vi "hough transform.vi"(10 "Threshold (0 - 255)":u8) -> (0 "error out":errorcluster)   [LabVIEW 2012]
uses:
  <vilib>/vision/Image Controls.llb/IMAQ Image.ctl
  <vilib>/vision/NI_Vision_Development_Module.lvlib
panel:
  out "Numeric 2":u32
  out "Numeric":u32
  out "Image 3":T1(plugin-control)
  out "Image 2":T1(plugin-control)
  in  "error in":errorcluster
  out "Image":T1
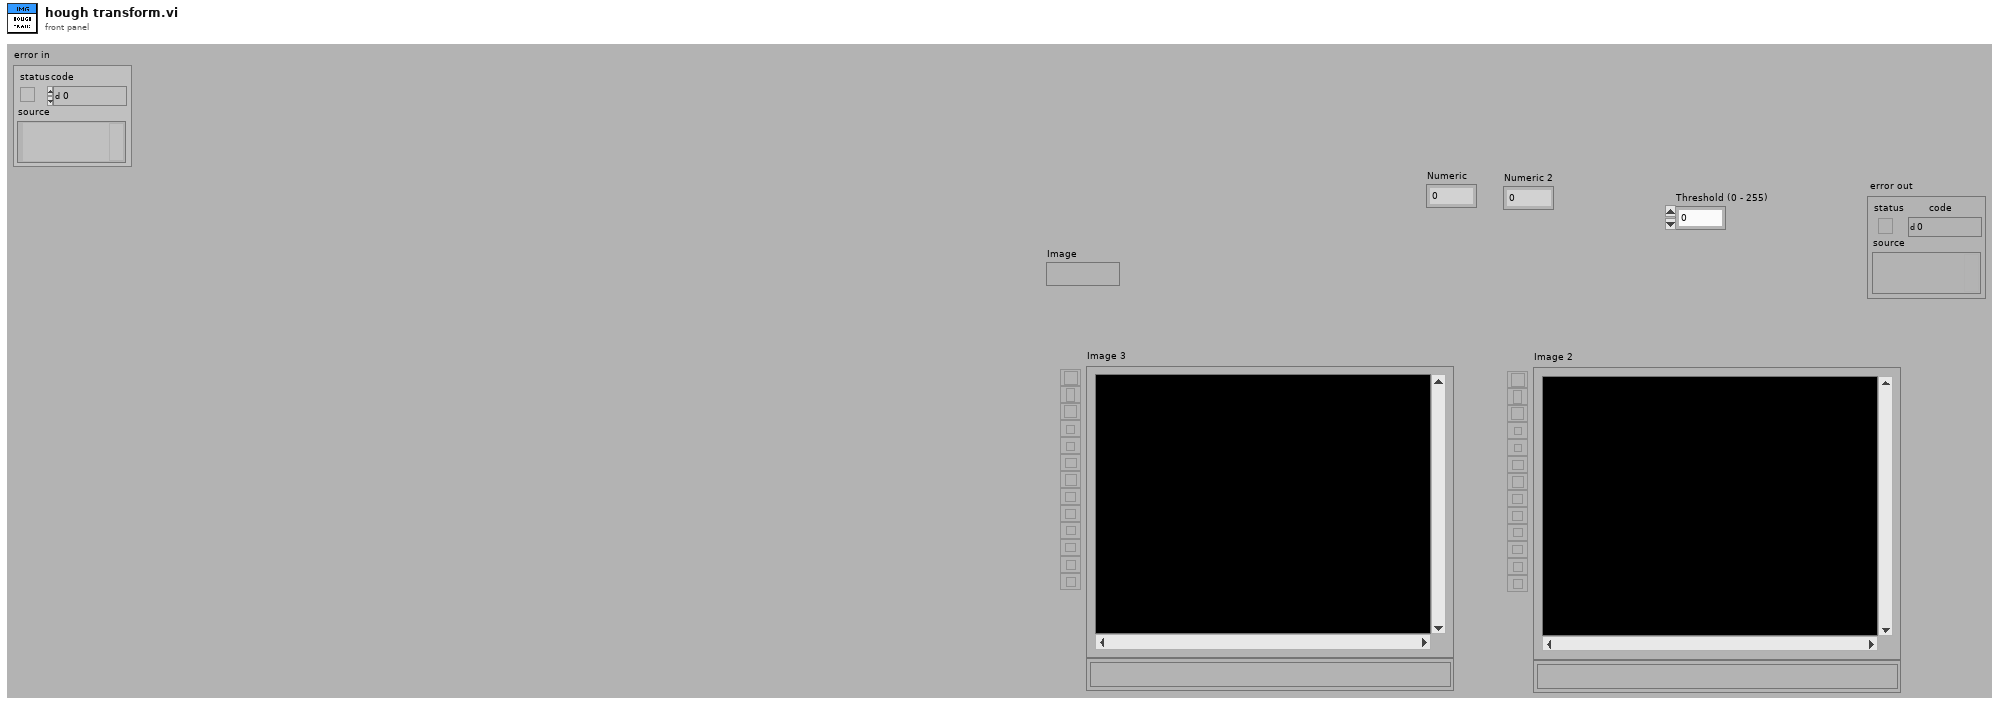
[diagram p1: front panel]
types:
  T1 = typedef "IMAQ Image.ctl" = refnum<image>
  T2 = typedef "Image Type" = u32
  T3 = enum32{"8 bits", "16 bits", "Float", "Complex", "RGB Chunky", "Compressed"}
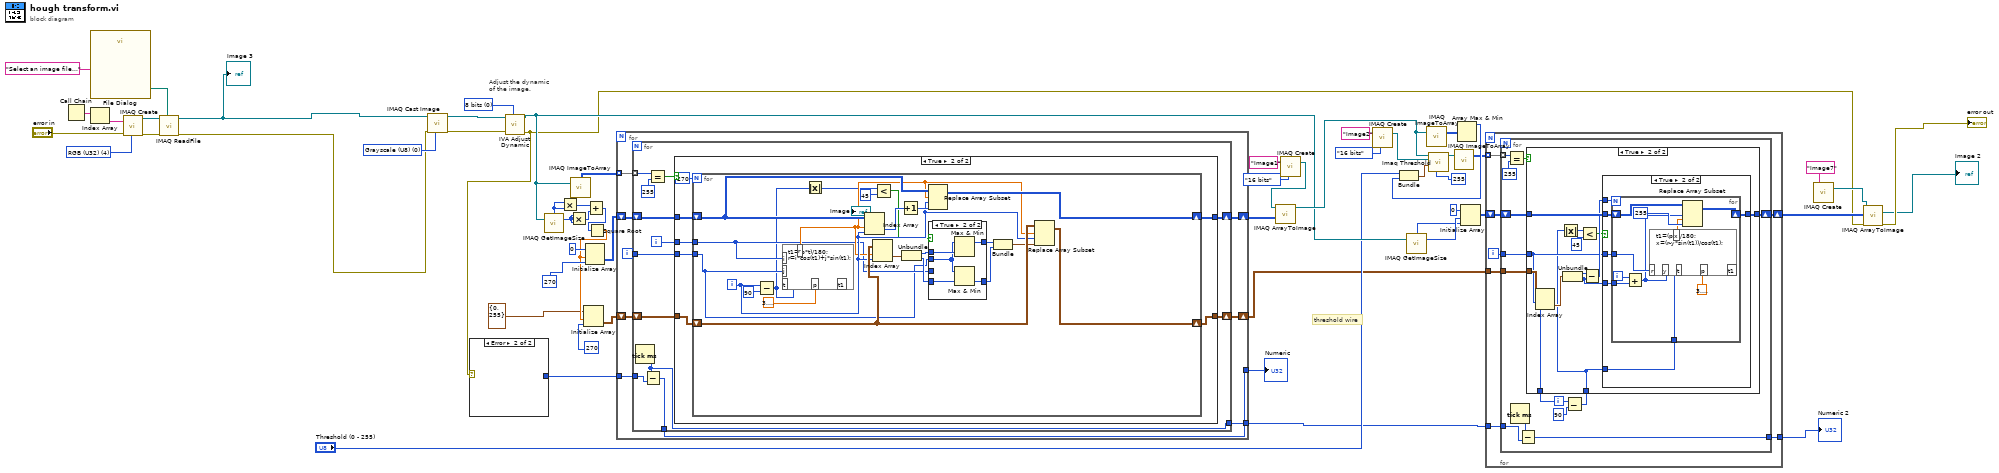
[diagram p0: block diagram]
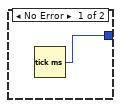
[diagram p2: hidden frame]
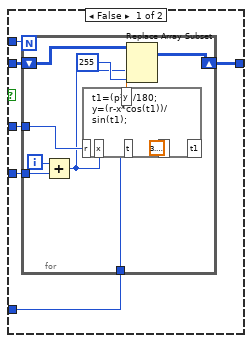
[diagram p4: hidden frame]
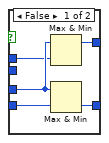
[diagram p6: hidden frame]
diagram:
  w10 = T2 4 items=["Grayscale (U8)", "Grayscale (I16)", "Grayscale (SGL)", "Complex (CSG)", "RGB (U32)", "HSL (U32)", "RGB (U64)", "Grayscale (U16)"] ("Image Type")
  w19 = T2 0 items=["Grayscale (U8)", "Grayscale (I16)", "Grayscale (SGL)", "Complex (CSG)", "RGB (U32)", "HSL (U32)", "RGB (U64)", "Grayscale (U16)"] ("Image Type")
  w24 = u32 0 items=["8 bits", "16 bits", "Float", "Complex", "RGB", "HSL"] ("Image Type")
  # "threshold wire"
  # "Adjust the dynamic\nof the image."
  n1 = Call Chain() -> (call chain=w14:string[])
  n2 = Index Array(array=w14) -> (element=w13:string)  [unwired: 1 in]
  n3 = call "File Dialog"("prompt"="Select an image file...") -> ("selected path"=w11:path)  [unwired: 6 in, 8 out]
  n4 = call "IMAQ Create"("Image Name"=w13, "Image Type"=w10, "error in (no error)"="error in") -> ("New Image"=w17:T1, "error out"=w16:errorcluster)  [unwired: 1 in, 1 out]
  n5 = call "IMAQ ReadFile"("File Path"=w11, "error in (no error)"=w16, "Image"=w17) -> ("error out"=w9:errorcluster, "Image Out"=w7:T1)  [unwired: 2 in, 5 out]
  "Image 3" <- w7
  n6 = call "IMAQ Cast Image"("Image Type"=w19, "error in (no error)"=w9, "Image Src"=w7) -> ("error out"=w21:errorcluster, "Image Dst Out"=w22:T1)  [unwired: 3 in, 4 out]
  n7 = call <vilib>:"IVA Adjust Dynamic.vi"("Image Type"=w24, "error in (no error)"=w21, "Image Src"=w22) -> ("error out"=w6:errorcluster, "Image Out"=w23:T1)  [unwired: 7 out]
  n8 = case shown="Error" w6 {
    tunnel: [w59 _] -> w5
    frame No Error {
      n9 = Tick Count (ms)() -> (millisecond timer value=w59:u32)
    }
    frame Error {
    }
  }
  n10 = call "IMAQ GetImageSize"("Image"=w23) -> ("Y Resolution"=w56:i32, "X Resolution"=w57:i32)  [unwired: 1 in, 3 out]
  n11 = Multiply(x=w57, y=w57) -> (x*y=w55:i32)
  n12 = Multiply(x=w56, y=w56) -> (x*y=w54:i32)
  n13 = call "IMAQ ImageToArray"("Image"=w23) -> ("Image Pixels (U8)"=w46:u8[][])  [unwired: 2 in, 5 out]
  n14 = Add(x=w55, y=w54) -> (x+y=w53:i32)
  n15 = Square Root(x=w53) -> (sqrt(x)=w44:dbl)
  n16 = Initialize Array(cluster{i32, i32} {0, 255}, w44, 270) -> (w43:cluster{i32, i32}[][])
  n17 = Initialize Array(0, w44, 270) -> (w50:i32[][])
  n18 = for {
    tunnel: w46 -> [w68] mode=indexing
    shift-right: [w66] -> w47
    shift-left: w50 -> [w65]
    shift-right: [w63] -> w4
    shift-left: w43 -> [w64]
    tunnel: w5 -> [w62]
    tunnel: [w61] -> w2
    tunnel: [w60] -> w3
    i -> [w67]
    n19 = for {
      tunnel: w68 -> [w80] mode=indexing
      tunnel: w67 -> [w76]
      shift-right: [w75] -> w66
      shift-left: w65 -> [w74]
      shift-right: [w72] -> w63
      shift-left: w64 -> [w73]
      tunnel: w62 -> [w71]
      tunnel: [w70] -> w61
      tunnel: [w69] -> w60
      i -> [w77]
      n20 = Tick Count (ms)() -> (millisecond timer value=w69:u32)
      n21 = Subtract(x=w69, y=w71) -> (x-y=w70:u32)
      n22 = Equal?(x=w80, y=u8 255) -> (x = y?=w78:bool)
      n23 = case shown="True" w78 {
        tunnel: w74 -> [w82 w86]
        tunnel: w77 -> [_ w88]
        tunnel: w76 -> [_ w87]
        tunnel: [w82 w85] -> w75
        tunnel: w73 -> [w81 w84]
        tunnel: [w81 w83] -> w72
        frame False {
        }
        frame True {
          n24 = for {
            N: 270 -> [_]
            tunnel: w88 -> [w99]
            tunnel: w87 -> [w95]
            shift-right: [w107] -> w85
            shift-left: w86 -> [w108]
            shift-right: [w106] -> w83
            shift-left: w84 -> [w105]
            i -> [w104]
            n25 = Subtract(x=w104, y=90) -> (x-y=w94:i32)
            n26 = formula code="t1=(p*t)/180;\nr=i*cos(t1)+j*sin(t1);"("t"=w94, "i"=w99, "j"=w95, "p"=3.141592653589793) -> ("r"=w103:dbl)  [unwired: 1 out]
            n27 = Absolute Value(x=w94) -> (abs(x)=w91:i32)
            n28 = Index Array(array=w108, index (row)=w103, index (col)=w104) -> (element=w110:i32)
            n29 = Index Array(array=w105, index (row)=w103, index (col)=w104) -> (element=w102:cluster{i32, i32})
            n30 = Less?(x=w91, y=45) -> (x < y?=w92:bool)
            n31 = Increment(x=w110) -> (x+1=w109:i32)
            n32 = Unbundle(w102) -> (w101:i32, w100:i32)
            n33 = Replace Array Subset(array=w108, new element=w109, index (row)=w103, index (col)=w104) -> (w107:i32[][])
            n34 = case shown="True" w92 {
              tunnel: [w116 w120] -> w97
              tunnel: [w115 w121] -> w98
              tunnel: w99 -> [w114 _]
              tunnel: w100 -> [w113 w118]
              tunnel: w101 -> [w112 w119]
              tunnel: w95 -> [_ w117]
              frame False {
                n35 = Max & Min(x=w114, y=w112) -> (max(x,y)=w115:i32)  [unwired: 1 out]
                n36 = Max & Min(x=w114, y=w113) -> (min(x,y)=w116:i32)  [unwired: 1 out]
              }
              frame True {
                n37 = Max & Min(x=w117, y=w119) -> (max(x,y)=w121:i32)  [unwired: 1 out]
                n38 = Max & Min(x=w117, y=w118) -> (min(x,y)=w120:i32)  [unwired: 1 out]
              }
            }
            n39 = Bundle(w98, w97) -> (w96:cluster{i32, i32})  [unwired: 1 out]
            n40 = Replace Array Subset(array=w105, new element=w96, index (row)=w103, index (col)=w104) -> (w106:cluster{i32, i32}[][])
          }
        }
      }
    }
  }
  "Numeric" <- w2
  n41 = call "IMAQ Create"("Image Name"="Image1", "Image Type"=T3."16 bits") -> ("New Image"=w49:T1)  [unwired: 2 in, 2 out]
  n42 = call "IMAQ ArrayToImage"("Image Pixels (I16)"=w47, "Image"=w49) -> ("Image Out"=w25:T1)  [unwired: 4 in, 5 out]
  n43 = call "IMAQ Create"("Image Name"="Image2", "Image Type"=T3."16 bits") -> ("New Image"=w39:T1)  [unwired: 2 in, 2 out]
  n44 = call "IMAQ GetImageSize"("Image"=w23) -> ("Y Resolution"=w30:i32, "X Resolution"=w29:i32)  [unwired: 1 in, 3 out]
  n45 = call "IMAQ ImageToArray"("Image"=w25) -> ("Image Pixels (I16)"=w37:i16[][])  [unwired: 2 in, 5 out]
  n46 = Array Max & Min(array=w37) -> (max value=w36:i16)  [unwired: 3 out]
  n47 = Bundle("Threshold (0 - 255)"="Threshold (0 - 255)", w36) -> (w41:cluster{"Threshold (0 - 255)":u8, i16})  [unwired: 1 out]
  n48 = call "Imaq Threshold"("Replace Value"=i16 255, "Range"=w41, "Image Dst"=w39, "Image Src"=w25) -> ("Image Dst Out"=w35:T1)  [unwired: 2 in, 5 out]
  n49 = call "IMAQ ImageToArray"("Image"=w35) -> ("Image Pixels (I16)"=w33:i16[][])  [unwired: 2 in, 5 out]
  n50 = Initialize Array(0, w30, w29) -> (w32:i32[][])
  n51 = for {
    tunnel: w33 -> [w128] mode=indexing
    shift-right: [w126] -> w26
    shift-left: w32 -> [w127]
    tunnel: w4 -> [w124]
    tunnel: w3 -> [w123]
    tunnel: [w122] -> w1
    i -> [w125]
    n52 = for {
      tunnel: w128 -> [w138] mode=indexing
      shift-right: [w139] -> w126
      shift-left: w127 -> [w140]
      tunnel: w125 -> [w134]
      tunnel: w124 -> [w133]
      tunnel: w123 -> [w130]
      tunnel: [w129] -> w122
      i -> [w132]
      n53 = Equal?(x=w138, y=i16 255) -> (x = y?=w137:bool)
      n54 = Tick Count (ms)() -> (millisecond timer value=w131:u32)
      n55 = Subtract(x=w131, y=w130) -> (x-y=w129:u32)
      n56 = Subtract(x=w132, y=90) -> (x-y=w135:i32)
      n57 = case shown="True" w137 {
        tunnel: w140 -> [w142 w155]
        tunnel: [w142 w154] -> w139
        tunnel: w134 -> [_ w147]
        tunnel: w135 -> [_ w146]
        tunnel: w133 -> [_ w151]
        tunnel: w132 -> [_ w150]
        frame False {
        }
        frame True {
          n58 = Index Array(array=w151, index (row)=w147, index (col)=w150) -> (element=w153:cluster{i32, i32})
          n59 = Absolute Value(x=w146) -> (abs(x)=w145:i32)
          n60 = Unbundle(w153) -> (w152:i32, w149:i32)
          n61 = Less?(x=w145, y=45) -> (x < y?=w144:bool)
          n62 = Subtract(x=w152, y=w149) -> (x-y=w148:i32)
          n63 = case shown="True" w144 {
            tunnel: w146 -> [w161 w173]
            tunnel: w147 -> [w160 w175]
            tunnel: w148 -> [w159 w177]
            tunnel: [w158 w172] -> w154
            tunnel: w155 -> [w157 w176]
            tunnel: w149 -> [w156 w174]
            frame False {
              n64 = for {
                N: w159 -> [_]
                shift-right: [w168] -> w158
                shift-left: w157 -> [w169]
                tunnel: w160 -> [w171]
                tunnel: w161 -> [w170]
                tunnel: w156 -> [w163]
                i -> [w164]
                n65 = Add(x=w164, y=w163) -> (x+y=w165:i32)
                n66 = formula code="t1=(p*t)/180;\ny=(r-x*cos(t1))/sin(t1);"("x"=w165, "r"=w171, "t"=w170, "p"=3.141592653589793) -> ("y"=w166:dbl)  [unwired: 1 out]
                n67 = Replace Array Subset(array=w169, new element=255, index (row)=w166, index (col)=w165) -> (w168:i32[][])
              }
            }
            frame True {
              n68 = for {
                N: w177 -> [_]
                shift-right: [w184] -> w172
                shift-left: w176 -> [w185]
                tunnel: w175 -> [w187]
                tunnel: w173 -> [w186]
                tunnel: w174 -> [w181]
                i -> [w182]
                n69 = Add(x=w182, y=w181) -> (x+y=w180:i32)
                n70 = formula code="t1=(p*t)/180;\nx=(r-y*sin(t1))/cos(t1);"("y"=w180, "r"=w187, "t"=w186, "p"=3.141592653589793) -> ("x"=w179:dbl)  [unwired: 1 out]
                n71 = Replace Array Subset(array=w185, new element=255, index (row)=w180, index (col)=w179) -> (w184:i32[][])
              }
            }
          }
        }
      }
    }
  }
  "Numeric 2" <- w1
  n72 = call "IMAQ Create"("Image Name"="Image7") -> ("New Image"=w27:T1)  [unwired: 3 in, 2 out]
  n73 = call "IMAQ ArrayToImage"("error in (no error)"=w6, "Image Pixels (U8)"=w26, "Image"=w27) -> ("error out"=→"error out":errorcluster, "Image Out"=→"Image 2":T1)  [unwired: 3 in, 4 out]
